vi "rollingAverage_IV.vi"(6 "Magnitude Averaging (no. Avgs.)":i32, 8 "785":T1, 9 "660":T3, 10 "532":T4, 11 "405":T5) -> (0 "785 Data":T2, 1 "660 Data":T7, 2 "532 Data":T8, 3 "405 Data":T6)   [LabVIEW 2011]
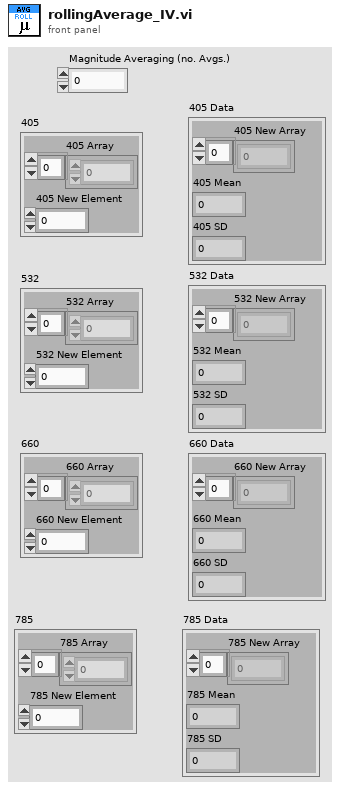
[diagram p1: front panel]
types:
  T1 = cluster{"785 Array":dbl[], "785 New Element":dbl}
  T2 = cluster{"785 New Array":dbl[], "785 Mean":dbl, "785 SD":dbl}
  T3 = cluster{"660 Array":dbl[], "660 New Element":dbl}
  T4 = cluster{"532 Array":dbl[], "532 New Element":dbl}
  T5 = cluster{"405 Array":dbl[], "405 New Element":dbl}
  T6 = cluster{"405 New Array":dbl[], "405 Mean":dbl, "405 SD":dbl}
  T7 = cluster{"660 New Array":dbl[], "660 Mean":dbl, "660 SD":dbl}
  T8 = cluster{"532 New Array":dbl[], "532 Mean":dbl, "532 SD":dbl}
  T9 = cluster{"New Array":dbl[], "mean":dbl, "standard deviation":dbl}
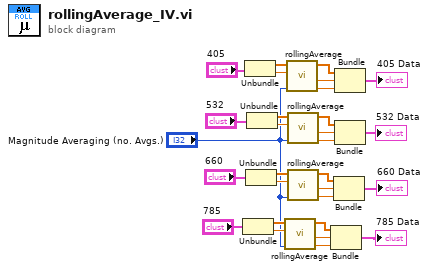
[diagram p0: block diagram]
diagram:
  n1 = Unbundle("785") -> ("785 Array"=w5:dbl[], "785 New Element"=w4:dbl)
  n2 = Unbundle("405") -> ("405 Array"=w24:dbl[], "405 New Element"=w25:dbl)
  n3 = Unbundle("660") -> ("660 Array"=w28:dbl[], "660 New Element"=w29:dbl)
  n4 = Unbundle("532") -> ("532 Array"=w26:dbl[], "532 New Element"=w27:dbl)
  n5 = call "rollingAverage.vi"("No Avg"="Magnitude Averaging (no. Avgs.)", "New Element"=w4, "Rolling Array"=w5) -> ("standard deviation"=w6:dbl, "mean"=w7:dbl, "New Array"=w8:dbl[])  [unwired: 6 in]
  n6 = call "rollingAverage.vi"("No Avg"="Magnitude Averaging (no. Avgs.)", "New Element"=w25, "Rolling Array"=w24) -> ("standard deviation"=w13:dbl, "mean"=w12:dbl, "New Array"=w23:dbl[])  [unwired: 6 in]
  n7 = call "rollingAverage.vi"("No Avg"="Magnitude Averaging (no. Avgs.)", "New Element"=w27, "Rolling Array"=w26) -> ("standard deviation"=w16:dbl, "mean"=w15:dbl, "New Array"=w14:dbl[])  [unwired: 6 in]
  n8 = call "rollingAverage.vi"("No Avg"="Magnitude Averaging (no. Avgs.)", "New Element"=w29, "Rolling Array"=w28) -> ("standard deviation"=w19:dbl, "mean"=w18:dbl, "New Array"=w17:dbl[])  [unwired: 6 in]
  n9 = Bundle("New Array"=w8, "mean"=w7, "standard deviation"=w6) -> (→"785 Data":T9)  [unwired: 1 in]
  n10 = Bundle("New Array"=w17, "mean"=w18, "standard deviation"=w19) -> (→"660 Data":T9)  [unwired: 1 in]
  n11 = Bundle("New Array"=w23, "mean"=w12, "standard deviation"=w13) -> (→"405 Data":T9)  [unwired: 1 in]
  n12 = Bundle("New Array"=w14, "mean"=w15, "standard deviation"=w16) -> (→"532 Data":T9)  [unwired: 1 in]
